vi "RTM - Export Configuration.vi"(8 "error in (no error)":errorcluster, 11 "Node Ptr":u64 format="%.0x") -> (0 "error out":errorcluster)   [LabVIEW 2019, in "UDP-Custom-Device System Explorer.lvlib"]
uses:
  UDP-Custom-Device System Explorer.lvlib
  <vilib>/NI/NI VeriStand Custom Device Import and Export Tool/ImportExport.lvlib
panel:
  in  "Tag":string
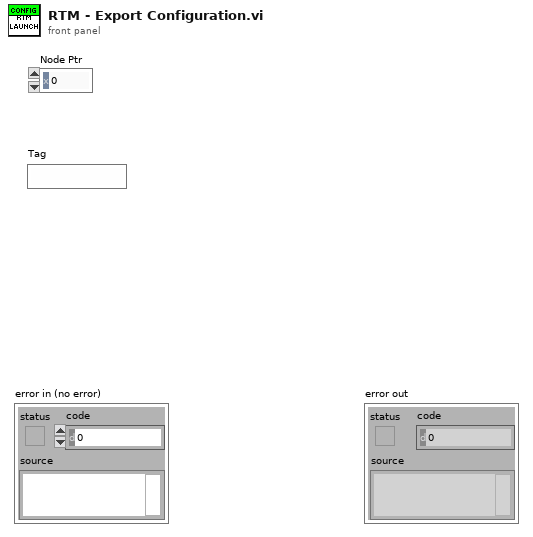
[diagram p1: front panel]
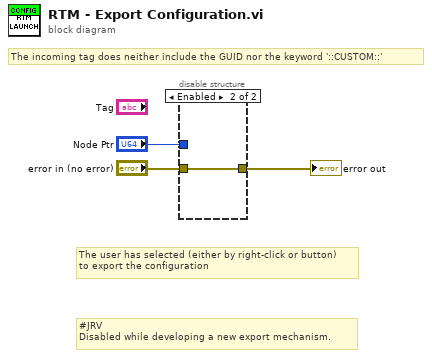
[diagram p0: block diagram]
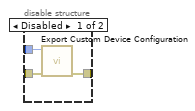
[diagram p2: hidden frame]
diagram:
  # "#JRV\nDisabled while developing a new export mechanism."
  # "The user has selected (either by right-click or button)\nto export the configuration"
  # "The incoming tag does neither include the GUID nor the keyword '::CUSTOM::'"
  n1 = disable-structure shown="Enabled" {
    disable-tunnel: [w6 w7] -> w3
    disable-tunnel: "error in (no error)" -> [w5 w7]
    disable-tunnel: "Node Ptr" -> [w4 _]
    frame Disabled {
      n2 = call <vilib>:"Export Custom Device Configuration.vi"("error in (no error)"=w5, "ID"=w4) -> ("error out"=w6:errorcluster)  [unwired: 8 in, 1 out]
    }
    frame Enabled {
    }
  }
  "error out" <- w3
